vi "bronkhorst_reg_simple.vi"(0 "SP":dbl caption="setpoint" step=0.01 format="%.2f", 1 "PV":dbl step=0.01 format="%.2f", 2 "PV_State":T2, 3 "Y":dbl step=0.01 format="%.2f", 4 "Y_State":T2, 6 "Y_Set":T4={"Y_HSw"=1, "Y_HSetState"=enum."auto", "Y_ASetState"=enum."auto", "Y_DSetState"=enum."auto"} {"Y_HSw" max=2 step=1}, 7 "controls Y":cluster{"Y_H":dbl, "Y_A":dbl, "Y_D":dbl} {"Y_H" format="%.2f"; "Y_D" format="%#_13g"; "Y_A" format="%#_13g"}, 8 "Z":T5, 9 "control param":T8={"proportional gain (Kc)"=1.0, "integral time (Ti, s)"=10.0, "derivative time (Td, s)"=1.0, "output high"=100.0, "output high start"=40.0, "output high stop"=40.0, "alr value"=0.0, "output low"=0.0, "output rate (EGU/s)"=5.0, "setpoint max"=100.0, "setpoint rate (EGU/min)"=10.0, "stop rate (EGU/min)"=5.0} {"setpoint max" format="%.2f"; "stop rate (EGU/min)" min=0.001 format="%.2f"; "setpoint rate (EGU/min)" min=0.001 format="%.2f"; "output high stop" format="%.2f"; "output high start" format="%.2f"; "output rate (EGU/s)" min=0.001 format="%.2f"; "output low" format="%.2f"; "alr value" format="%.2f"; "output high" format="%.2f"; "derivative time (Td, s)" format="%.3f"; "integral time (Ti, s)" format="%.3f"; "proportional gain (Kc)" format="%.3f"}, 10 "XB24 (F)":bool, 11 "Start":bool) -> (14 "Y_State":T6={"Y_Source"=enum."local disabled", "Y_SetState"=enum."auto", "SP_Set"=0.0, "SP"=0.0, "PV"=0.0, "PV_State"={"code"=0, "visible"=FALSE, "color"=0}, "Y_preSet"=0.0, "Y_Set"=0.0, "Y"=0.0, "Y_State"={"code"=0, "visible"=FALSE, "color"=0}, "YB"=FALSE} {"Y" format="%.2f"; "Y_preSet" format="%.2f"; "SP" step=0.01 format="%.2f"; "Y_Set" format="%.2f"; "PV" step=0.01 format="%.2f"; "SP_Set" step=0.01 format="%.2f"}, 15 "Y":dbl format="%.2f", 17 "T":u32, 18 "End":bool)   [LabVIEW 2019, in "control.lvlib"]
uses:
  control.lvlib
  ctl/control param.ctl
  ctl/Y.ctl
  ctl/Y_source.ctl
  ctl/Y_state.ctl
  Inputs/Ctl/Parameter State short.ctl
  ctl/Z_State.ctl
  ctl/Y_Lim_State.ctl
  PID Output Rate Limiter.vi
  PID Timing Estimation.vi
  Inputs/Inputs.lvlib
panel:
  out "SpLim_State":T1=enum."increase"
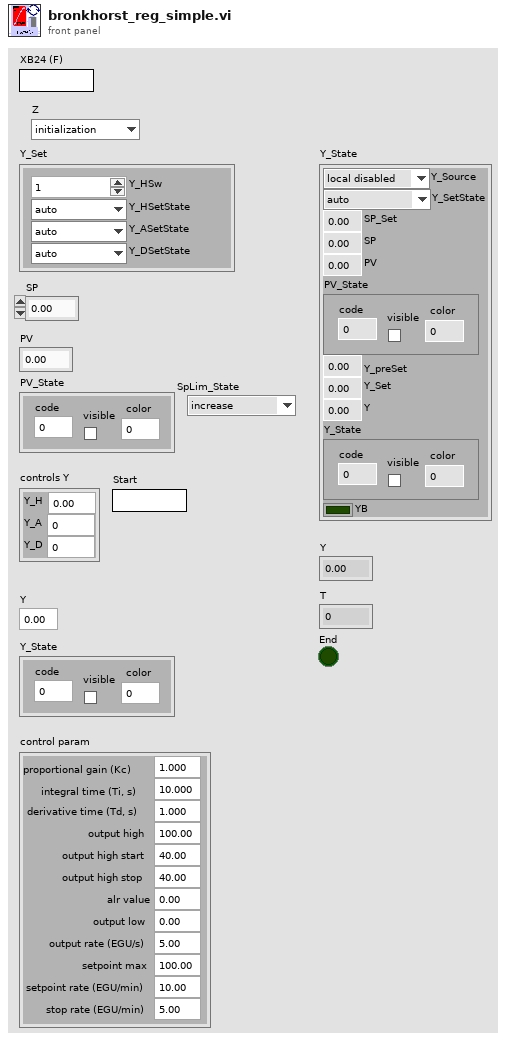
[diagram p1: front panel]
types:
  T1 = typedef "Y_Lim_State.ctl" = enum8{"initialization", "alarm", "stop", "decrease", "increase"}
  T2 = typedef "Inputs.lvlib/Parameter State short.ctl" = cluster{"code":i32, "visible":bool, "color":u32}
  T3 = typedef "control.lvlib/Y_state.ctl" = enum8{"initialize", "alarm", "min", "stop", "hand", "auto", "max"}
  T4 = cluster{"Y_HSw":u32, "Y_HSetState":T3, "Y_ASetState":T3, "Y_DSetState":T3}
  T5 = typedef "control.lvlib/Z_State.ctl" = enum8{"initialization", "alarm", "disabled", "not ready", "stop ready", "reserv", "switched off", "reserv2", "switched on", "check", "on min", "decrease out", "on", "increase out", "on max"}
  T6 = typedef "control.lvlib/Y.ctl" = cluster{"Y_Source":T7, "Y_SetState":T3, "SP_Set":dbl, "SP":dbl, "PV":dbl, "PV_State":T2, "Y_preSet":dbl, "Y_Set":dbl, "Y":dbl, "Y_State":T2, "YB":bool}
  T7 = typedef "control.lvlib/Y_source.ctl" = enum8{"initialize", "local disabled", "local hand", "hand", "auto", "dist"}
  T8 = typedef "control.lvlib/control param.ctl" = cluster{"proportional gain (Kc)":dbl, "integral time (Ti, s)":dbl, "derivative time (Td, s)":dbl, "output high":dbl, "output high start":dbl, "output high stop":dbl, "alr value":dbl, "output low":dbl, "output rate (EGU/s)":dbl, "setpoint max":dbl, "setpoint rate (EGU/min)":dbl, "stop rate (EGU/min)":dbl}
  T9 = enum8{"alarm", "min", "stop", "hand", "auto", "max"}
  T10 = cluster{"output high":dbl, "alr value":dbl, "output low":dbl, "output rate (EGU/s)":dbl}
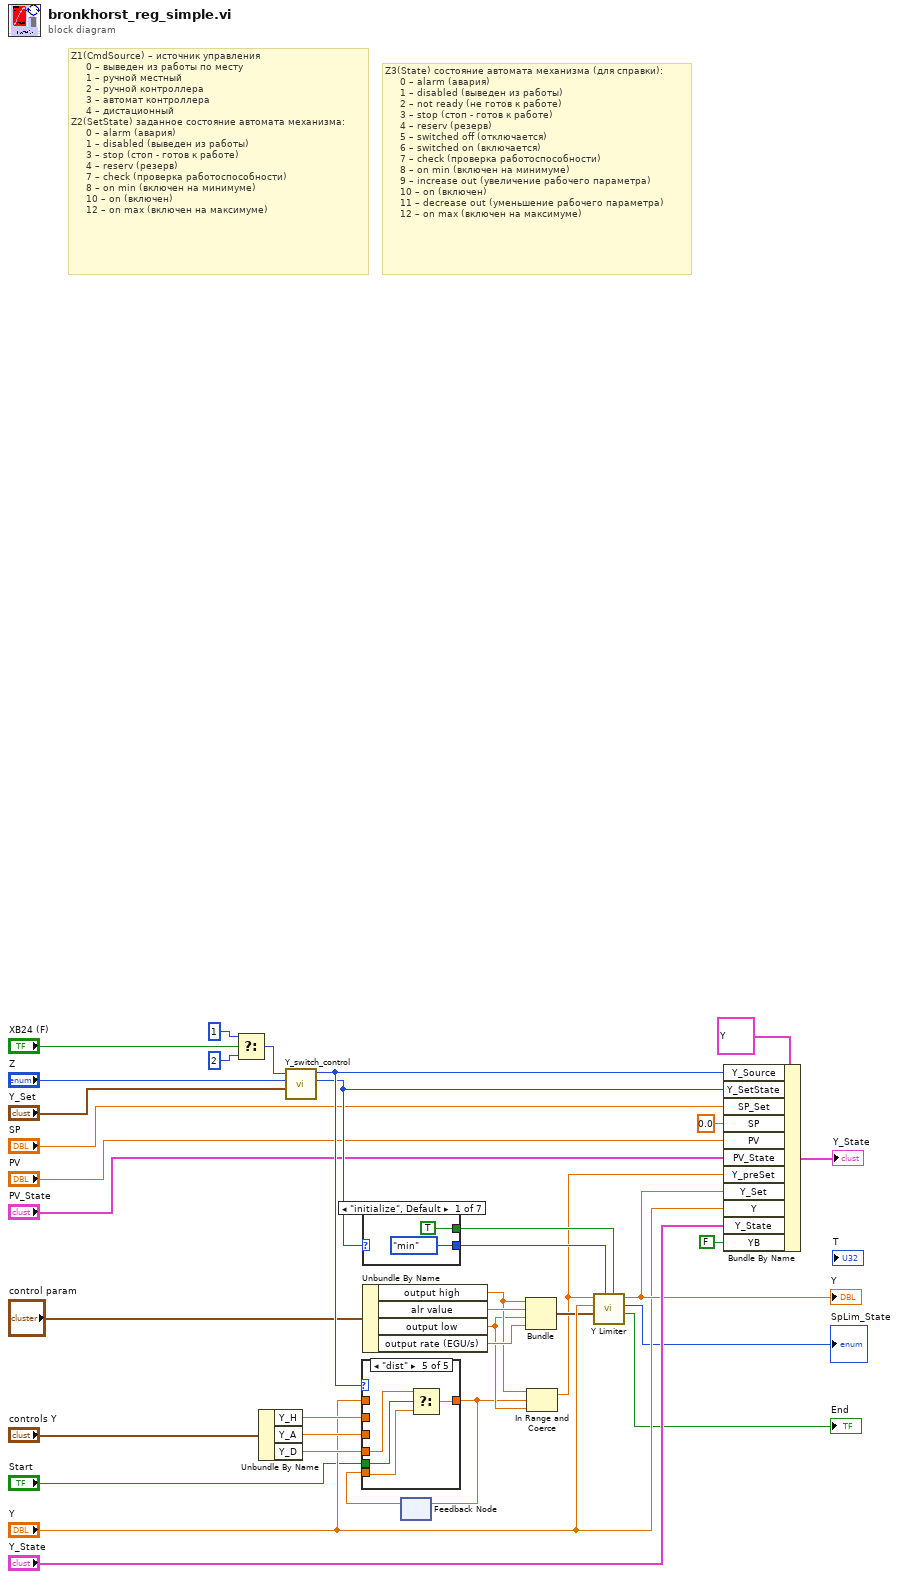
[diagram p0: block diagram]
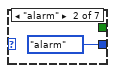
[diagram p2: hidden frame]
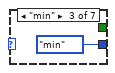
[diagram p3: hidden frame]
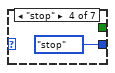
[diagram p4: hidden frame]
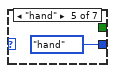
[diagram p5: hidden frame]
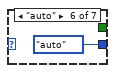
[diagram p6: hidden frame]
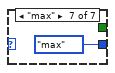
[diagram p7: hidden frame]
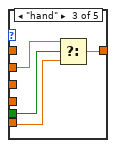
[diagram p10: hidden frame]
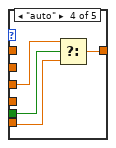
[diagram p11: hidden frame]
diagram:
  # "Z1(CmdSource) – источник управления\n     0 – выведен из работы по месту\n     1 – ручной местный\n     2 – ручной контроллера\n     3 – автомат контроллера\n     4 – дистационный\nZ2(SetState) заданное состояние автомата механизма:\n     0 – alarm (авария)\n     1 – disabled (выведен из работы)\n     3 – stop (стоп - готов к работе)\n     4 – reserv (резерв)\n     7 – check (проверка работоспособности)\n     8 – on min (включен на минимуме)\n     10 – on (включен)\n     12 – on max (включен на максимуме)"
  # "Z3(State) состояние автомата механизма (для справки):\n     0 – alarm (авария)\n     1 – disabled (выведен из работы)\n     2 – not ready (не готов к работе)\n     3 – stop (стоп - готов к работе)\n     4 – reserv (резерв)\n     5 – switched off (отключается)\n     6 – switched on (включается)\n     7 – check (проверка работоспособности)\n     8 – on min (включен на минимуме)\n     9 – increase out (увеличение рабочего параметра)\n     10 – on (включен)\n     11 – decrease out (уменьшение рабочего параметра)\n     12 – on max (включен на максимуме)"
  n1 = Select(t=u32 1, s="XB24 (F)", f=u32 2 ("Y_HSw")) -> (s? t:f=w32:u32)
  n2 = Unbundle By Name("controls Y") -> ("Y_H"=w19:dbl, "Y_A"=w36:dbl, "Y_D"=w35:dbl)
  n3 = call "Y_switch_control.vi"("Y"="Y_Set", "Z_State"="Z", "Y_LSw (2-auto)"=w32) -> ("Y_SetState"=w29:T3, "Y_Source"=w30:T7)  [unwired: 7 in]
  n4 = case shown="\"initialize\", Default" w29 {
    tunnel: [T9."min" ("X1(SetState)") T9."alarm" ("X1(SetState)") T9."min" ("X1(SetState)") T9."stop" ("X1(SetState)") T9."hand" ("X1(SetState)") T9."auto" ("X1(SetState)") T9."max" ("X1(SetState)")] -> w15
    tunnel: [TRUE _ _ _ _ _ _] -> w17
    frame "initialize", Default {
    }
    frame "alarm" {
    }
    frame "min" {
    }
    frame "stop" {
    }
    frame "hand" {
    }
    frame "auto" {
    }
    frame "max" {
    }
  }
  n5 = Unbundle By Name("control param") -> ("output high"=w8:dbl, "alr value"=w12:dbl, "output low"=w6:dbl, "output rate (EGU/s)"=w11:dbl)
  n6 = feedback #1() -> (w4:dbl)  [unwired: 1 in]
  n7 = case shown="\"dist\"" w30 {
    tunnel: w19 -> [_ _ w47 _ _]
    tunnel: "Y" -> [w45 w46 _ _ _]
    tunnel: w35 -> [_ _ _ _ w57]
    tunnel: [w45 w46 w50 w54 w58] -> w5
    tunnel: w36 -> [_ _ _ w51 _]
    tunnel: w4 -> [_ _ w49 w53 w56]
    tunnel: "Start" -> [_ _ w48 w52 w55]
    frame "local disabled", Default {
    }
    frame "local hand" {
    }
    frame "hand" {
      n8 = Select(t=w47, s=w48, f=w49) -> (s? t:f=w50:dbl)
    }
    frame "auto" {
      n9 = Select(t=w51, s=w52, f=w53) -> (s? t:f=w54:dbl)
    }
    frame "dist" {
      n10 = Select(t=w57, s=w55, f=w56) -> (s? t:f=w58:dbl)
    }
  }
  n11 = feedback-in #1(w5) -> ()
  n12 = Bundle("output high"=w8, "alr value"=w12, "output low"=w6, "output rate (EGU/s)"=w11) -> (w10:T10)  [unwired: 1 in]
  n13 = In Range and Coerce(upper limit=w8, x=w5, lower limit=w6) -> (coerced(x)=w7:dbl)  [unwired: 1 out]
  n14 = call "Y Limiter.vi"("reinitialize? (F)"=w17, "X1(SetState)"=w15, "Y param"=w10, "Y (NaN)"="Y", "Y_Set"=w7) -> ("End"=→"End":bool, "SpLim_State"=→"SpLim_State":T1, "output"=w18:dbl)  [unwired: 4 in]
  "Y" <- w18
  n15 = Bundle By Name(cluster=T6 {"Y_Source"=enum."local disabled", "Y_SetState"=enum."auto", "SP_Set"=0.0, "SP"=0.0, "PV"=0.0, "PV_State"={"code"=0, "visible"=FALSE, "color"=0}, "Y_preSet"=0.0, "Y_Set"=0.0, "Y"=0.0, "Y_State"={"code"=0, "visible"=FALSE, "color"=0}, "YB"=FALSE} ("Y_State"), "Y_Source"=w30, "Y_SetState"=w29, "SP_Set"="SP", "SP"=0.0, "PV"="PV", "PV_State"="PV_State", "Y_preSet"=w7, "Y_Set"=w18, "Y"="Y", "Y_State"="Y_State", "YB"=FALSE) -> (→"Y_State":T6)
